vi "write.vi"(8 "error in (no error)":errorcluster, 9 "bytes to write":i32, 10 "data":string, 11 "file descriptor in":i32) -> (0 "error out":errorcluster, 1 "bytes written":i32, 3 "file descriptor out":i32)   [LabVIEW 2013, in "Pipes.lvlib"]
uses:
  Pipes.lvlib
  Controls/functions.ctl
  <vilib>/NI/NI Linux RT Errno/Linux Errno.lvlib
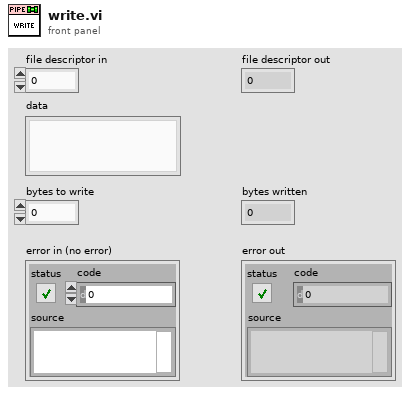
[diagram p1: front panel]
types:
  T1 = typedef "Pipes.lvlib/functions.ctl" = enum16{"unspecified", "mkfifo", "open", "read", "write", "close", "unlink"}
  T2 = typedef "Linux Errno.lvlib/errno.ctl" = enum16{"NO ERROR", "EPERM", "ENOENT", "ESRCH", "EINTR", "EIO", "ENXIO", "E2BIG", "ENOEXEC", "EBADF", "ECHILD", "EAGAIN", "ENOMEM", "EACCES", "EFAULT", "ENOTBLK", "EBUSY", "EEXIST", "EXDEV", "ENODEV", "ENOTDIR", "EISDIR", "EINVAL", "ENFILE", "EMFILE", "ENOTTY", "ETXTBSY", "EFBIG", "ENOSPC", "ESPIPE", "EROFS", "EMLINK", "EPIPE", "EDOM", "ERANGE", "EDADLK", "ENAMETOOLONG", "ENOLCK", "ENOSYS", "ENOTEMPTY", "ELOOP", "EWOULDBLOCK", "ENOMSG", "EIDRM", "ECHRNG", "EL2NSYNC", "EL3HLT", "EL3RST", "ELNRNG", "EUNATCH", "ENOCSI", "EL2HLT", "EBADE", "EBADR", "EXFULL", "ENOANO", "EBADRQC", "EBADSLT", "EDEADLOCK", "EBFONT", "ENOSTR", "ENODATA", "ETIME", "ENOSR", "ENONET", "ENOPKG", "EREMOTE", "ENOLINK", "EADV", "ESRMNT", "ECOMM", "EPROTO", "EMULTIHOP", "EDOTDOT", "EBADMSG", "EOVERFLOW", "ENOTUNIQ", "EBADFD", "EREMCHG", "ELIBACC", "ELIBBAD", "ELIBSCN", "ELIBMAX", "ELIBEXEC", "ELISEQ", "ERESTART", "ESTRPIPE", "EUSERS", "ENOTSOCK", "EDESTADDRREQ", "EMSGSIZE", "EPROTOTYPE", "ENOPROTOOPT", "EPROTONOSUPPORT", "ESOCKTNOSUPPORT", "EOPNOTSUPP", "EPFNOSUPPORT", "EAFNOSUPPORT", "EADDRINUSE", "EADDRNOTAVAIL", "ENETDOWN", "ENETUNREACH", "ENETRESET", "ECONNABORTED", "ECONNRESET", "ENOBUFS", "EISCONN", "ENOTCONN", "ESHUTDOWN", "ETOOMANYREFS", "ETIMEDOUT", "ECONNREFUSED", "EHOSTDOWN", "EHOSTUNREACH", "EALREADY", "EINPROGRESS", "ESTALE", "EUCLEAN", "ENOTNAM", "ENAVAIL", "EISNAM", "EREMOTEIO", "EDQUOT", "ENOMEDIUM", "EMEDIUMTYPE", "ECANCELED", "ENOKEY", "EKEYEXPIRED", "EKEYREVOKED", "EKEYREJECTED", "EOWNERDEAD", "ENOTRECOVERABLE", "ERFKILL", "EHWPOISON", "UNDEFINED"}
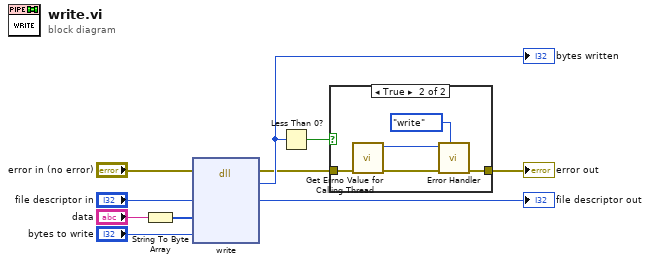
[diagram p0: block diagram]
diagram:
  n1 = String To Byte Array(string="data") -> (unsigned byte array=w4:u8[])
  n2 = dll-call lib="LabVIEW" fn="write"(error in="error in (no error)", "fd"="file descriptor in", "buf"=w4, "count"="bytes to write") -> (error out=w3:errorcluster, "return"=w7:i32, "fd"=→"file descriptor out":i32)  [unwired: 4 in, 1 out]
  "bytes written" <- w7
  n3 = Less Than 0?(x=w7) -> (x < 0?=w2:bool)
  n4 = case shown="True" w2 {
    tunnel: w3 -> [w11 w16]
    tunnel: [w11 w14] -> w1
    frame False {
    }
    frame True {
      n5 = call <vilib>:"Get Errno Value for Calling Thread.vi"("error in (no error)"=w16) -> ("error out"=w12:errorcluster, "errno"=w13:T2)  [unwired: 9 in]
      n6 = call "Error Handler.vi"("function (unspecified)"=functions."write", "error in (no error)"=w12, "errno"=w13) -> ("error out"=w14:errorcluster)  [unwired: 8 in]
    }
  }
  "error out" <- w1
